vi "HSLtoRGB.vi"(9 "Lightness":dbl, 10 "Saturation":dbl=1.0, 11 "Hue":dbl) -> (1 "Blue":u8, 2 "Green":u8, 3 "Red":u8)   [LabVIEW 2026]
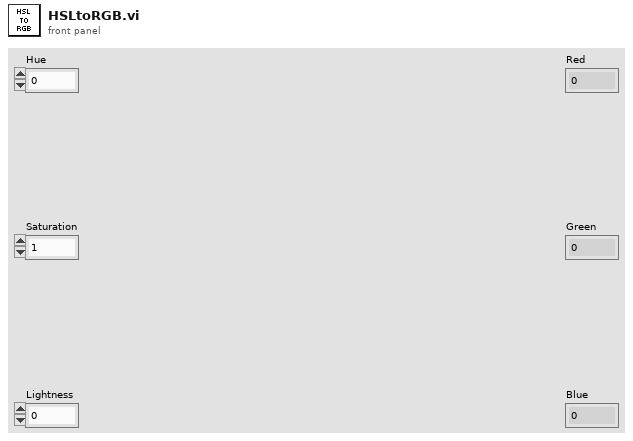
[diagram p1: front panel]
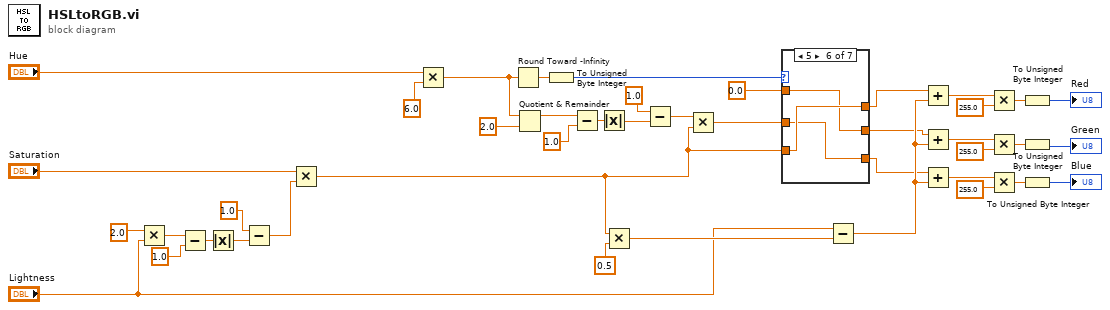
[diagram p0: block diagram]
diagram:
  n1 = Multiply(x=2.0 ("y"), y="Lightness") -> (x*y=w42:dbl)
  n2 = Subtract(x=w42, y=1.0) -> (x-y=w40:dbl)
  n3 = Absolute Value(x=w40) -> (abs(x)=w39:dbl)
  n4 = Subtract(x=1.0, y=w39) -> (x-y=w13:dbl)
  n5 = Multiply(x="Saturation", y=w13) -> (x*y=w4:dbl)
  n6 = Multiply(x="Hue", y=6.0) -> (x*y=w25:dbl)
  n7 = Round Toward -Infinity(1:w25) -> (0:w35:dbl)
  n8 = Quotient & Remainder(x=w25, y=2.0) -> (x-y*floor(x/y)=w23:dbl)  [unwired: 1 out]
  n9 = To Unsigned Byte Integer(number=w35) -> (unsigned 8bit integer=w7:u8)
  n10 = Subtract(x=w23, y=1.0) -> (x-y=w21:dbl)
  n11 = Absolute Value(x=w21) -> (abs(x)=w20:dbl)
  n12 = Multiply(x=w4, y=0.5) -> (x*y=w11:dbl)
  n13 = Subtract(x=1.0, y=w20) -> (x-y=w18:dbl)
  n14 = Multiply(x=w18, y=w4) -> (x*y=w5:dbl)
  n15 = case shown="5" w7 {
    tunnel: w4 -> [w45 w47 w50 w52 w55 w60 _]
    tunnel: w5 -> [w44 w48 w49 w53 w57 w58 _]
    tunnel: 0.0 -> [w43 w46 w51 w54 w56 w59 w61]
    tunnel: [w45 w48 w51 w54 w57 w60 w61] -> w1
    tunnel: [w44 w47 w50 w53 w56 w59 w61] -> w2
    tunnel: [w43 w46 w49 w52 w55 w58 w61] -> w3
    frame 0 {
    }
    frame 1 {
    }
    frame 2 {
    }
    frame 3 {
    }
    frame 4 {
    }
    frame 5 {
    }
    frame Default {
    }
  }
  n16 = Subtract(x="Lightness", y=w11) -> (x-y=w10:dbl)
  n17 = Add(x=w1, y=w10) -> (x+y=w26:dbl)
  n18 = Add(x=w2, y=w10) -> (x+y=w27:dbl)
  n19 = Add(x=w3, y=w10) -> (x+y=w28:dbl)
  n20 = Multiply(x=w26, y=255.0) -> (x*y=w33:dbl)
  n21 = Multiply(x=w27, y=255.0) -> (x*y=w32:dbl)
  n22 = Multiply(x=w28, y=255.0) -> (x*y=w30:dbl)
  n23 = To Unsigned Byte Integer(number=w33) -> (unsigned 8bit integer=→"Red":u8)
  n24 = To Unsigned Byte Integer(number=w32) -> (unsigned 8bit integer=→"Green":u8)
  n25 = To Unsigned Byte Integer(number=w30) -> (unsigned 8bit integer=→"Blue":u8)
